vi "PID_CLIENTE.vi"() -> ()   [LabVIEW 2025]
panel:
  in  "INDICADORES DE SINTONIA":bool
  out "kd":dbl(slide) scale=0.0..10.0
  out "ki":dbl(slide) scale=0.0..10.0
  out "kp":dbl(slide) scale=0.0..10.0
  in  "porta":dbl
  in  "kd":dbl
  in  "ki":dbl
  in  "kp":dbl
  out "Numeric":dbl
  in  "ON/ OFF":bool
  out "DOSAGEM":string
  out "bytes escritos":i32
  out "açao de controle":string
  out "tipo de dosagem":string
  in  "Setpoint":dbl(slide) scale=0.8..1.4
  out "dado enviado para o servidor":string
  out "indicador de set point":string
  out "indicador de densidade":string
  in  "parametro a":dbl format="%#_13g"
  in  "parametro b":dbl format="%#_13g"
  in  "parametro c":dbl format="%#_13g"
  out "densidadeA":dbl
  out "SINAL DE CONTROLE AGUA":dbl(graph)
  out "Q1":dbl
  in  "barita g/s":dbl(slide) scale=0.0..1000.0
  out "densidadeB":dbl
  out "SINAL DE CONTROLE BARITA":dbl(graph)
  in  "A":dbl=0.1 format="%#_13g"
  in  "B":dbl=0.2 format="%#_13g"
  in  "C":dbl format="%#_13g"
  out "W2":dbl
  in  "agua cm3/s":dbl(slide) scale=0.0..500.0
  out "DENSIDADE E SET POINT":cluster{dbl, "Setpoint":dbl}(graph)
  # "MODELO/ÁGUA"
  # "MODELO/BARITA"
  # "SINTONIA"
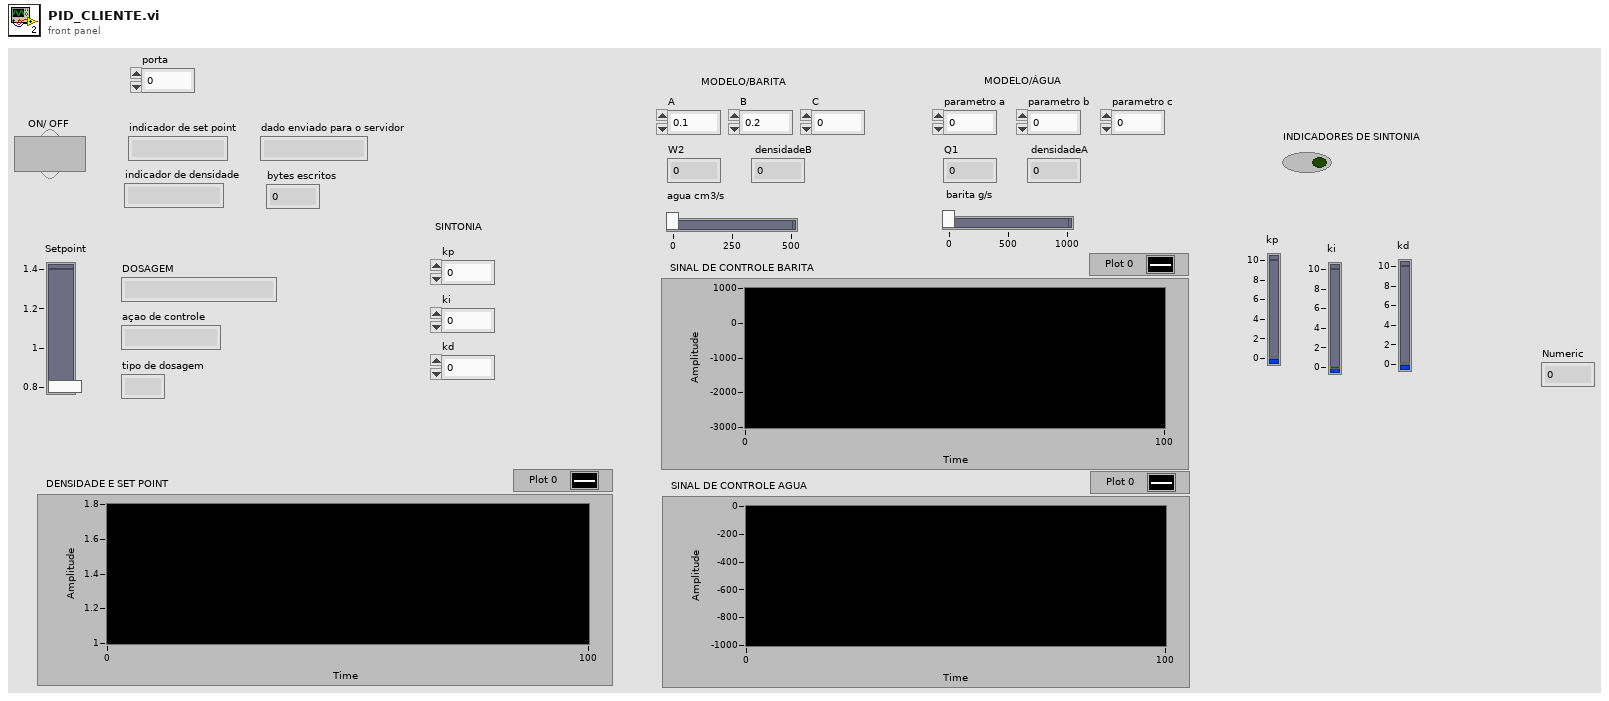
[diagram p1: front panel]
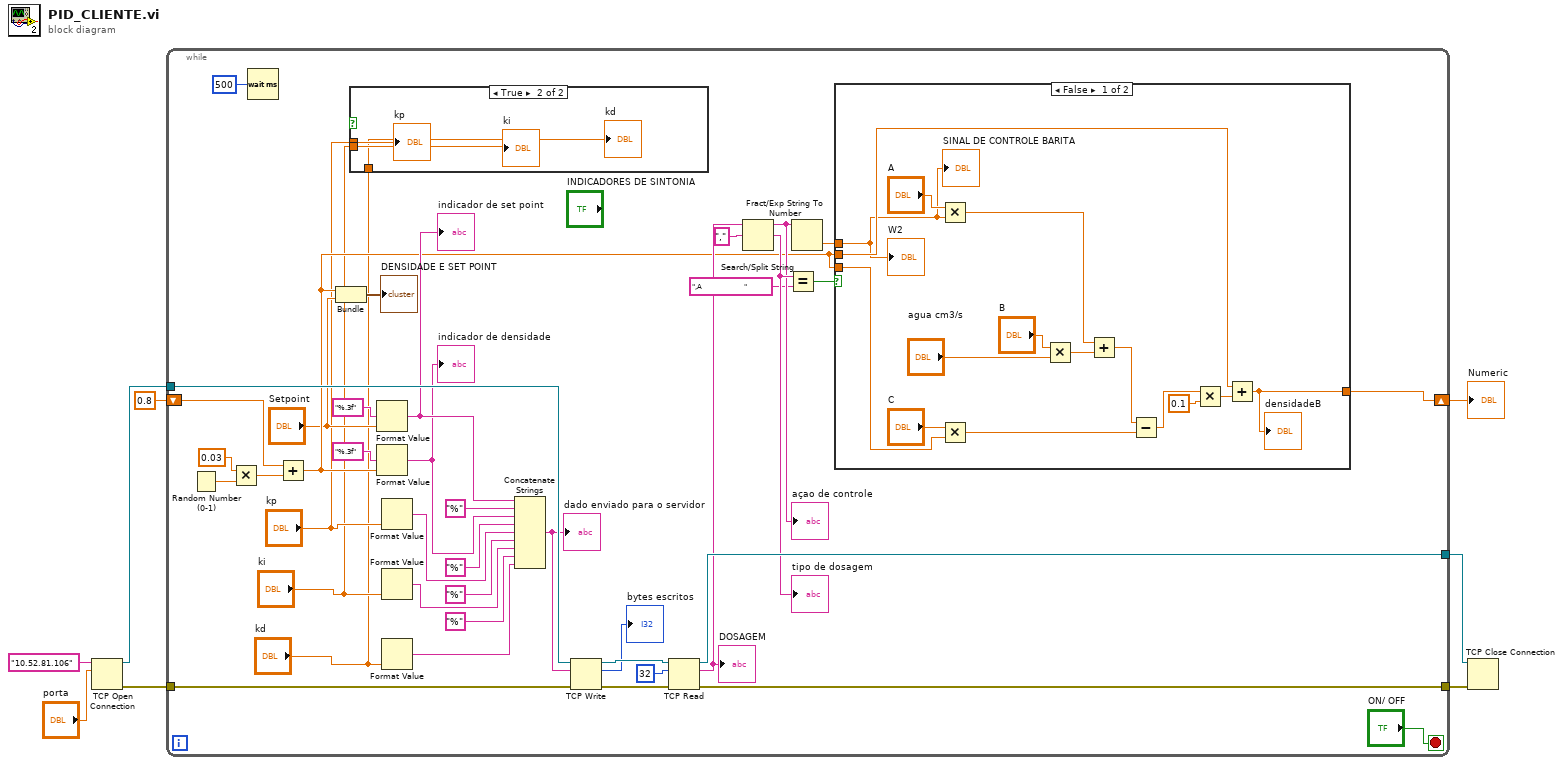
[diagram p0: block diagram]
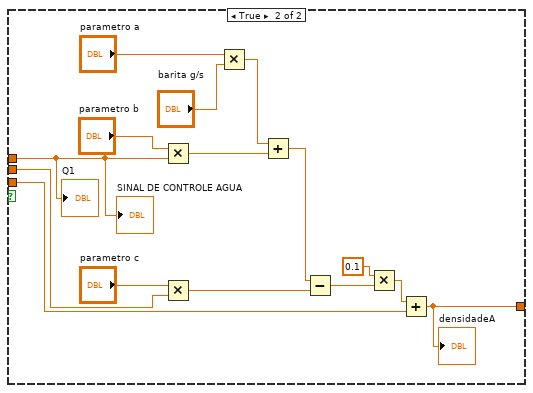
[diagram p3: hidden frame]
diagram:
  n1 = TCP Open Connection(address="10.52.81.106", remote port or service name="porta") -> (connection ID=w8:refnum<k5>, error out=w7:errorcluster)  [unwired: 3 in]
  n2 = while {
    tunnel: w8 -> [w47]
    tunnel: w7 -> [w46]
    tunnel: [w43] -> w6
    tunnel: [w42] -> w5
    shift-right: [w29] -> w3
    shift-left: 0.8 -> [w26]
    stop <- "ON/ OFF" stop-if-true
    n3 = Random Number (0-1)() -> (number: 0 to 1=w25:dbl)
    n4 = Multiply(x=0.03, y=w25) -> (x*y=w24:dbl)
    n5 = Wait (ms)(milliseconds to wait=500) -> ()  [unwired: 1 out]
    n6 = Add(x=w26, y=w24) -> (x+y=w22:dbl)
    n7 = Bundle(w22, "Setpoint"="Setpoint") -> (→"DENSIDADE E SET POINT":cluster{dbl, "Setpoint":dbl})  [unwired: 1 in]
    n8 = case shown="True" w12 {
      tunnel: "kp" -> [_ w52]
      tunnel: "ki" -> [_ w51]
      tunnel: "kd" -> [_ w50]
      frame False {
      }
      frame True {
        "kp" <- w52
        "ki" <- w51
        "kd" <- w50
      }
    }
    n9 = Format Value(format string="%.3f", value (0)="Setpoint") -> (output string=w33:string)  [unwired: 1 in]
    "indicador de set point" <- w33
    n10 = Format Value(format string="%.3f", value (0)=w22) -> (output string=w32:string)  [unwired: 1 in]
    "indicador de densidade" <- w32
    n11 = Format Value(value (0)="kp") -> (output string=w15:string)  [unwired: 2 in]
    n12 = Format Value(value (0)="ki") -> (output string=w14:string)  [unwired: 2 in]
    n13 = Format Value(value (0)="kd") -> (output string=w13:string)  [unwired: 2 in]
    n14 = Concatenate Strings(w33, "%" ("string"), w32, "%" ("string"), w15, "%" ("string"), w14, "%" ("string"), w13) -> (w36:string)
    "dado enviado para o servidor" <- w36
    n15 = TCP Write(connection ID=w47, data in=w36, error in (no error)=w46) -> (connection ID out=w45:refnum<k5>, bytes written=→"bytes escritos":i32, error out=w44:errorcluster)  [unwired: 1 in]
    n16 = TCP Read(connection ID=w45, bytes to read=32, error in (no error)=w44) -> (connection ID out=w42:refnum<k5>, data out=w39:string, error out=w43:errorcluster)  [unwired: 2 in]
    "DOSAGEM" <- w39
    n17 = Search/Split String(string=w39, search string/char (-)=",") -> (substring before match=w28:string, match + rest of string=w31:string)  [unwired: 1 in, 1 out]
    "açao de controle" <- w28
    "tipo de dosagem" <- w31
    n18 = Equal?(x=w31, y=",A                     ") -> (x = y?=w30:bool)
    n19 = Fract/Exp String To Number(string=w28) -> (number=w27:dbl)  [unwired: 3 in, 1 out]
    n20 = case shown="False" w30 {
      tunnel: [w61 w70] -> w29
      tunnel: w27 -> [w53 w68]
      tunnel: w22 -> [w58 w71]
      tunnel: w22 -> [w55 w77]
      frame False {
        n21 = Multiply(x="A", y=w53) -> (x*y=w63:dbl)
        n22 = Multiply(x="C", y=w58) -> (x*y=w57:dbl)
        n23 = Multiply(x="B", y="agua cm3/s") -> (x*y=w62:dbl)
        n24 = Add(x=w63, y=w62) -> (x+y=w60:dbl)
        n25 = Subtract(x=w60, y=w57) -> (x-y=w56:dbl)
        n26 = Multiply(x=w56, y=0.1) -> (x*y=w64:dbl)
        n27 = Add(x=w55, y=w64) -> (x+y=w61:dbl)
        "densidadeB" <- w61
        "SINAL DE CONTROLE BARITA" <- w53
        "W2" <- w53
      }
      frame True {
        n28 = Multiply(x="parametro b", y=w68) -> (x*y=w79:dbl)
        n29 = Multiply(x="parametro c", y=w77) -> (x*y=w76:dbl)
        n30 = Multiply(x="parametro a", y="barita g/s") -> (x*y=w80:dbl)
        n31 = Add(x=w80, y=w79) -> (x+y=w75:dbl)
        n32 = Subtract(x=w75, y=w76) -> (x-y=w74:dbl)
        n33 = Multiply(x=0.1, y=w74) -> (x*y=w72:dbl)
        n34 = Add(x=w72, y=w71) -> (x+y=w70:dbl)
        "densidadeA" <- w70
        "SINAL DE CONTROLE AGUA" <- w68
        "Q1" <- w68
      }
    }
  }
  "Numeric" <- w3
  n35 = TCP Close Connection(connection ID=w5, error in (no error)=w6) -> ()  [unwired: 1 in, 2 out]
